vi "FFT-Presentation.vi"() -> ()   [LabVIEW 2014]
doc: "Use this template to build a VI to use as a subVI."
uses:
  <vilib>/vision/NI_Vision_Development_Module.lvlib
panel:
  out "MagF":T1(plugin-control)
  out "IF(u,v)I":T1(plugin-control)
  out "Src":T1(plugin-control)
  # ":: MVi Framework V1.0 ::\nAuthor:Gaoke Yang\nEmail: gaoke.yang@yahoo.com\nWeb: www.mvicontrol.com\nCopyright (C) 2015, MVI Technologies All Rights Reserved"
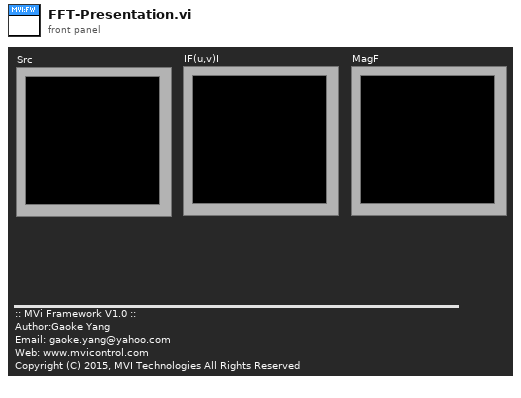
[diagram p1: front panel]
types:
  T1 = typedef "IMAQ Image.ctl" = refnum<image>
  T2 = enum32{"Real", "Imaginary", "Magnitude", "Phase"}
  T3 = typedef "Image Type" = u32
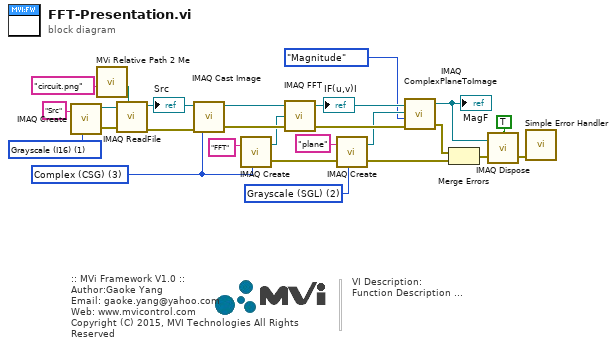
[diagram p0: block diagram]
diagram:
  w10 = T3 1 items=["Grayscale (U8)", "Grayscale (I16)", "Grayscale (SGL)", "Complex (CSG)", "RGB (U32)", "HSL (U32)", "RGB (U64)", "Grayscale (U16)"] ("Image Type")
  w16 = T3 2 items=["Grayscale (U8)", "Grayscale (I16)", "Grayscale (SGL)", "Complex (CSG)", "RGB (U32)", "HSL (U32)", "RGB (U64)", "Grayscale (U16)"] ("Image Type")
  w4 = T3 3 items=["Grayscale (U8)", "Grayscale (I16)", "Grayscale (SGL)", "Complex (CSG)", "RGB (U32)", "HSL (U32)", "RGB (U64)", "Grayscale (U16)"] ("Image Type")
  # "VI Description:\nFunction Description ..."
  # ":: MVi Framework V1.0 ::\nAuthor:Gaoke Yang\nEmail: gaoke.yang@yahoo.com\nWeb: www.mvicontrol.com\nCopyright (C) 2015, MVI Technologies All Rights Reserved"
  n1 = call "IMAQ Create"("Image Name"="Src" ("name or relative path"), "Image Type"=w10) -> ("New Image"=w23:T1, "error out"=w22:errorcluster)  [unwired: 2 in, 1 out]
  n2 = call "MVi Relative Path 2 Me.vi"("Relative Path"="circuit.png" ("name or relative path")) -> ("Appended Dir"=w19:path)  [unwired: 5 in, 1 out]
  n3 = call "IMAQ ReadFile"("File Path"=w19, "error in (no error)"=w22, "Image"=w23) -> ("error out"=w14:errorcluster, "Image Out"=w18:T1)  [unwired: 4 in, 3 out]
  "Src" <- w18
  n4 = call "IMAQ Cast Image"("Image Type"=w4, "error in (no error)"=w14, "Image Src"=w18) -> ("error out"=w13:errorcluster, "Image Dst Out"=w12:T1)  [unwired: 7 in]
  n5 = call "IMAQ Create"("Image Name"="FFT" ("name or relative path"), "Image Type"=w4) -> ("New Image"=w11:T1, "error out"=w7:errorcluster)  [unwired: 2 in, 1 out]
  n6 = call "IMAQ FFT"("error in (no error)"=w13, "Image Dst"=w11, "Image Src"=w12) -> ("error out"=w8:errorcluster, "Image Dst Out"=w9:T1)  [unwired: 1 in]
  "IF(u,v)I" <- w9
  n7 = call "IMAQ Create"("Image Name"="plane" ("name or relative path"), "Image Type"=w16, "error in (no error)"=w7) -> ("New Image"=w6:T1, "error out"=w3:errorcluster)  [unwired: 1 in, 1 out]
  n8 = call "IMAQ ComplexPlaneToImage"("error in (no error)"=w8, "Plane"=T2."Magnitude", "Image Dst"=w6, "Image Src"=w9) -> ("error out"=w2:errorcluster, "Image Dst Out"=w1:T1)  [unwired: 1 in]
  "MagF" <- w1
  n9 = Merge Errors(w2, w3) -> (w17:errorcluster)
  n10 = call "IMAQ Dispose"("All Images? (No)"=TRUE, "Image"=w1, "error in (no error)"=w17) -> ("error out"=w24:errorcluster)  [unwired: 3 out]
  n11 = call <vilib>:"Simple Error Handler.vi"("error in (no error)"=w24) -> ()  [unwired: 1 in, 8 out]
